vi "CD Read Engine_Simulate Records.vi"(8 "error in (no error)":errorcluster) -> (0 "error out":errorcluster, 3 "Record []":T1[](array[typedef]) {"type" format="%04x"; "activity" format="%04x"; "error" format="%04x"; "cwd1" format="%04x"; "cwd2" format="%04x"; "swd1" format="%04x"; "swd2" format="%04x"; "data" format="%04x"})   [LabVIEW 2017, in "Ballard MIL-1553 Engine.lvlib"]
uses:
  Ballard MIL-1553 Engine.lvlib
  <instrlib>/BTICardLib/Public/Controls/1553 Record.ctl
  <instrlib>/BTICardLib/BTICardLV.lvlib
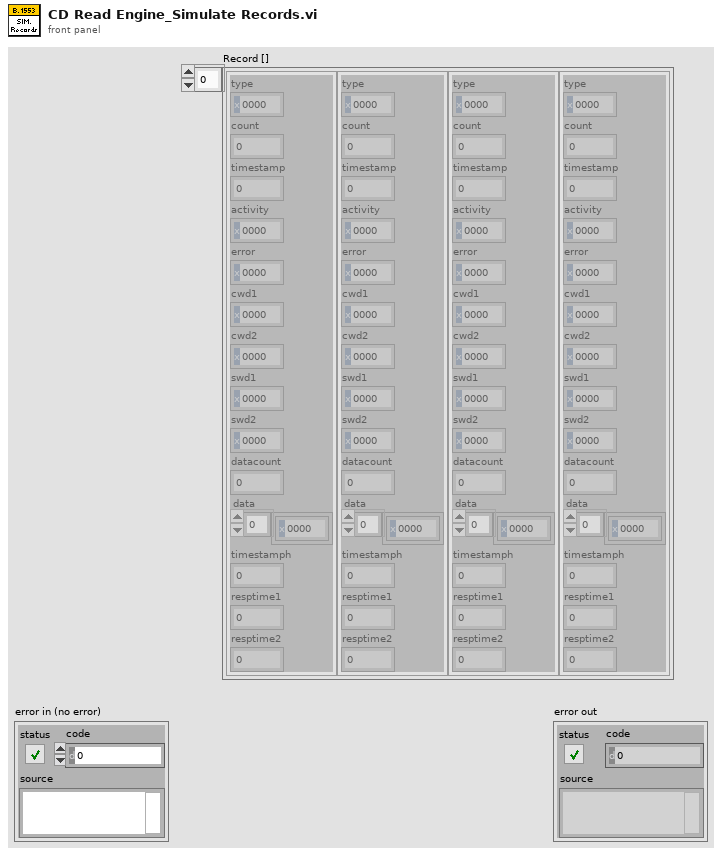
[diagram p1: front panel]
types:
  T1 = typedef "BTICardLV.lvlib/1553 Record.ctl" = cluster{"type":u16, "count":u16, "timestamp":u32, "activity":u16, "error":u16, "cwd1":u16, "cwd2":u16, "swd1":u16, "swd2":u16, "datacount":u16, "data":u16[], "timestamph":u32, "resptime1":u16, "resptime2":u16}
  T2 = cluster{"type":u16, "count":i32, "timestamp":u32, "activity":i32, "error":u16, "cwd1":i32, "cwd2":i32, "swd1":i32, "swd2":i32, "datacount":i32, "data":u16[], "timestamph":u32, "resptime1":u16, "resptime2":u16}
  T3 = cluster{"type":u16, "count":i32, "timestamp":u32, "activity":i32, "error":u16, "cwd1":i32, "cwd2":i32, "swd1":i32, "swd2":i32, "datacount":i32, "data":u16[], "timestamph":u32, "resptime1":u16, "resptime2":u16}[]
  T4 = cluster{"type":u16, "count":i32, "timestamp":u32, "activity":i32, "error":u16, "cwd1":i32, "cwd2":i32, "swd1":u16, "swd2":i32, "datacount":i32, "data":u16[], "timestamph":u32, "resptime1":u16, "resptime2":u16}
  T5 = cluster{"type":u16, "count":i32, "timestamp":u32, "activity":i32, "error":u16, "cwd1":i32, "cwd2":i32, "swd1":u16, "swd2":i32, "datacount":i32, "data":u16[], "timestamph":u32, "resptime1":u16, "resptime2":u16}[]
  T6 = cluster{"type":u16, "count":i32, "timestamp":u32, "activity":i32, "error":i32, "cwd1":i32, "cwd2":i32, "swd1":u16, "swd2":i32, "datacount":i32, "data":u16[], "timestamph":u32, "resptime1":u16, "resptime2":u16}
  T7 = cluster{"type":u16, "count":i32, "timestamp":u32, "activity":i32, "error":i32, "cwd1":i32, "cwd2":i32, "swd1":u16, "swd2":i32, "datacount":i32, "data":u16[], "timestamph":u32, "resptime1":u16, "resptime2":u16}[]
  T8 = cluster{"type":u16, "count":i32, "timestamp":u32, "activity":i32, "error":i32, "cwd1":i32, "cwd2":i32, "swd1":i32, "swd2":i32, "datacount":i32, "data":u16[], "timestamph":u32, "resptime1":u16, "resptime2":u16}[]
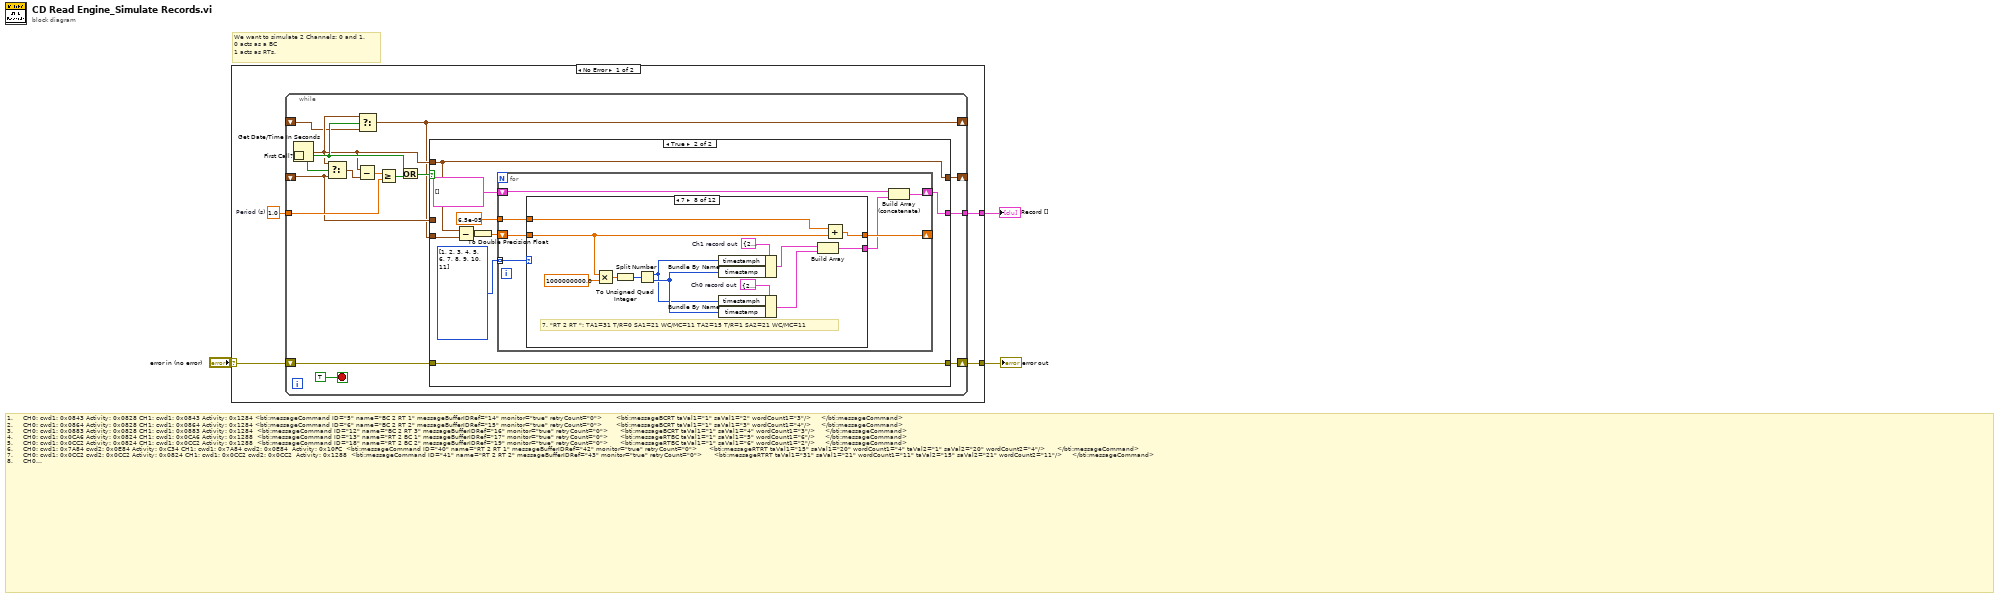
[diagram p0: block diagram]
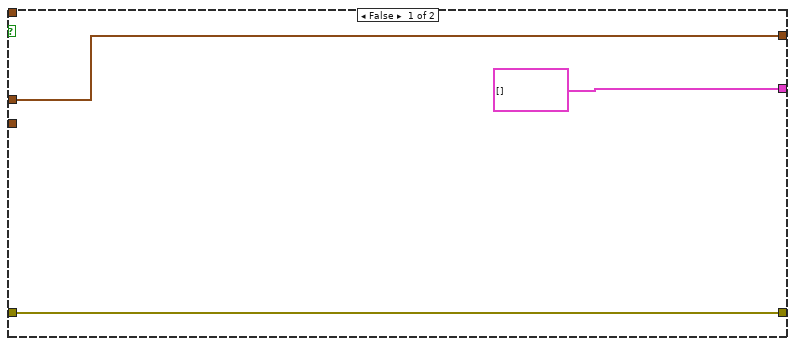
[diagram p2: hidden frame]
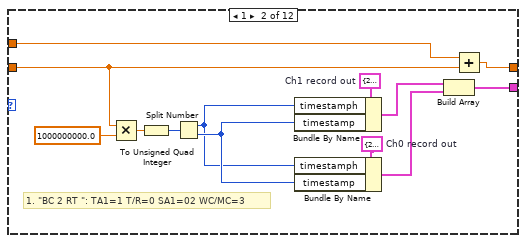
[diagram p4: hidden frame]
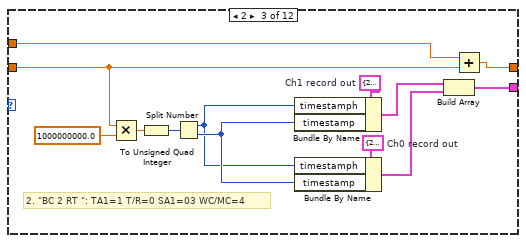
[diagram p5: hidden frame]
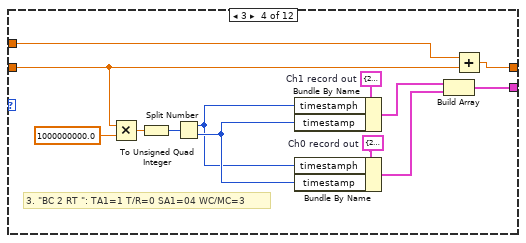
[diagram p6: hidden frame]
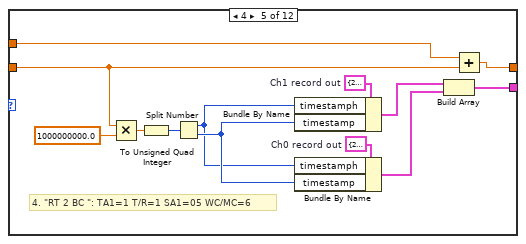
[diagram p7: hidden frame]
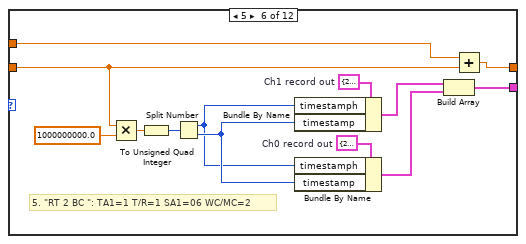
[diagram p8: hidden frame]
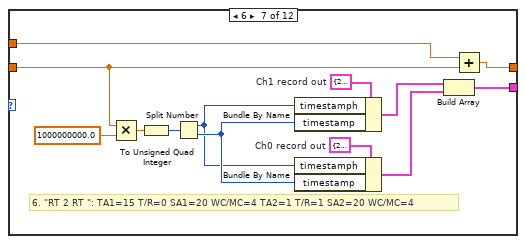
[diagram p9: hidden frame]
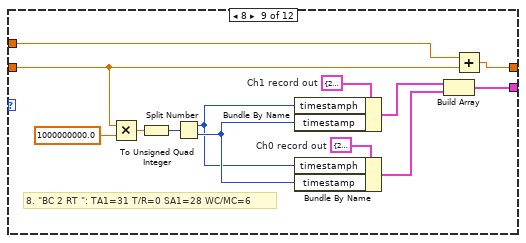
[diagram p10: hidden frame]
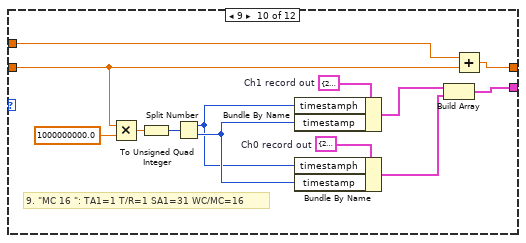
[diagram p11: hidden frame]
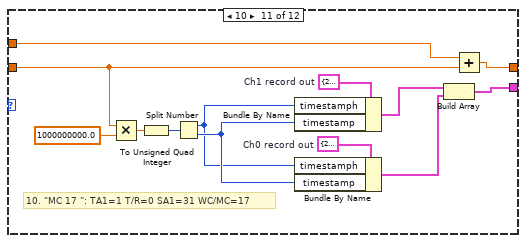
[diagram p12: hidden frame]
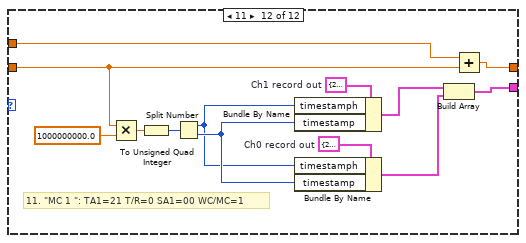
[diagram p13: hidden frame]
diagram:
  # "1.\t\t\t\t\tCH0: cwd1: 0x0843 Activity: 0x0828 CH1: cwd1: 0x0843 Activity: 0x1284 <bti:messageCommand ID=\"5\" name=\"BC 2 RT 1\" messageBufferIDRef=\"14\" monitor=\"true\" retryCount=\"0\"> \t\t\t\t\t\t<bti:messageBCRT taVal1=\"1\" saVal1=\"2\" wordCount1=\"3\"/>\t\t\t\t\t</bti:messageCommand>\n2.\t\t\t\t CH0: cwd1: 0x0864 Activity: 0x0828 CH1: cwd1: 0x0864 Activity: 0x1284 <bti:messageCommand ID=\"6\" name=\"BC 2 RT 2\" messageBufferIDRef=\"15\" monitor=\"true\" retryCount=\"0\"> \t\t\t\t\t\t<bti:messageBCRT taVal1=\"1\" saVal1=\"3\" wordCount1=\"4\"/>\t\t\t\t\t</bti:messageCommand>\n3.\t\t\t\t CH0: cwd1: 0x0883 Activity: 0x0828 CH1: cwd1: 0x0883 Activity: 0x1284 \t<bti:messageCommand ID=\"12\" name=\"BC 2 RT 3\" messageBufferIDRef=\"16\" monitor=\"true\" retryCount=\"0\">\t\t\t\t\t\t<bti:messageBCRT taVal1=\"1\" saVal1=\"4\" wordCount1=\"3\"/>\t\t\t\t\t</bti:messageCommand>\n4.\t\t\t\t\tCH0: cwd1: 0x0CA6 Activity: 0x0824 CH1: cwd1: 0x0CA6 Activity: 0x1288 \t<bti:messageCommand ID=\"13\" name=\"RT 2 BC 1\" messageBufferIDRef=\"17\" monitor=\"true\" retryCount=\"0\">\t\t\t\t\t\t<bti:messageRTBC taVal1=\"1\" saVal1=\"5\" wordCount1=\"6\"/>\t\t\t\t\t</bti:messageCommand>\n5.\t\t\t\t\tCH0: cwd1: 0x0CC2 Activity: 0x0824 CH1: cwd1: 0x0CC2 Activity: 0x1288 \t<bti:messageCommand ID=\"18\" name=\"RT 2 BC 2\" messageBufferIDRef=\"19\" monitor=\"true\" retryCount=\"0\">\t\t\t\t\t\t<bti:messageRTBC taVal1=\"1\" saVal1=\"6\" wordCount1=\"2\"/>\t\t\t\t\t</bti:messageCommand>\n6.\t\t\t\t\tCH0: cwd1: 0x7A84 cwd2: 0x0E84 Activity: 0xC34 CH1: cwd1: 0x7A84 cwd2: 0x0E84  Activity: 0x10FC \t<bti:messageCommand ID=\"40\" name=\"RT 2 RT 1\" messageBufferIDRef=\"42\" monitor=\"true\" retryCount=\"0\">\t\t\t\t\t\t<bti:messageRTRT taVal1=\"15\" saVal1=\"20\" wordCount1=\"4\" taVal2=\"1\" saVal2=\"20\" wordCount2=\"4\"/> \t\t\t\t\t</bti:messageCommand>\n7.\t\t\t\t\tCH0: cwd1: 0x0CC2 cwd2: 0x0CC2 Activity: 0x0824 CH1: cwd1: 0x0CC2 cwd2: 0x0CC2  Activity: 0x1288 \t<bti:messageCommand ID=\"41\" name=\"RT 2 RT 2\" messageBufferIDRef=\"43\" monitor=\"true\" retryCount=\"0\">\t\t\t\t\t\t<bti:messageRTRT taVal1=\"31\" saVal1=\"21\" wordCount1=\"11\" taVal2=\"15\" saVal2=\"21\" wordCount2=\"11\"/>\t\t\t\t\t</bti:messageCommand>\n8.\t\t\t\t\tCH0: cwd1: 0xFB86 Activity: 0x0808 CH1: cwd1: 0xFB86 Activity: 0x1084 <bti:messageCommand ID=\"44\" name=\"BC 2 RT 4\" messageBufferIDRef=\"45\" monitor=\"true\" retryCount=\"0\">\t\t\t\t\t\t<bti:messageBCRT taVal1=\"31\" saVal1=\"28\" wordCount1=\"6\"/> \t\t\t\t\t</bti:messageCommand>\n9.\t\t\t\t\tCH0: cwd1: 0x0FE1 Activity: 0x820 CH1: cwd1: 0x0FE1 Activity: 0x1280 <bti:messageCommand ID=\"50\" name=\"MC 16\" messageBufferIDRef=\"53\" monitor=\"true\" retryCount=\"0\">\t\t\t\t\t\t<bti:messageMC taVal1=\"1\" saVal1=\"31\" modeCodeNumber=\"16\" direction=\"Tx\"/>\t\t\t\t\t</bti:messageCommand>\n10.\t\t\tCH0: cwd1: 0x0BF1 Activity: 0x0828 CH1: cwd1: 0x0BF1 Activity: 0x1284\t\t<bti:messageCommand ID=\"51\" name=\"MC 17\" messageBufferIDRef=\"54\" monitor=\"true\" retryCount=\"0\">\t\t\t\t\t\t<bti:messageMC taVal1=\"1\" saVal1=\"31\" modeCodeNumber=\"17\" direction=\"Rx\"/>\t\t\t\t\t</bti:messageCommand>\n11.\t\t\tCH0: cwd1: 0xA801 Activity: 0x1280 CH1: cwd1:A801 0x Activity: 0x0820\t\t<bti:messageCommand ID=\"52\" name=\"MC 1\" messageBufferIDRef=\"55\" monitor=\"true\" retryCount=\"0\">\t\t\t\t\t\t<bti:messageMC taVal1=\"21\" saVal1=\"00\" modeCodeNumber=\"1\" direction=\"Rx\"/>\t\t\t\t\t</bti:messageCommand>"
  # "We want to simulate 2 Channels: 0 and 1.\n0 acts as a BC\n1 acts as RTs."
  n1 = case shown="No Error" "error in (no error)" {
    selector: "error in (no error)" -> [w7 w186]
    tunnel: [w6 w186] -> w2
    tunnel: [w4 _] -> w1
    frame No Error {
      w5 = 1.0  # Period (s)
      n2 = while {
        shift-right: [w15] -> w6
        shift-left: w7 -> [w16]
        shift-right: [w12] -> _
        shift-left: _ -> [w13]
        tunnel: w5 -> [w19]
        tunnel: [w14] -> w4
        shift-right: [w8] -> _
        shift-left: _ -> [w9]
        stop <- TRUE stop-if-true
        n3 = First Call?() -> (First Call?: T/F=w11:bool)
        n4 = Get Date/Time In Seconds() -> (seconds since 1Jan1904=w10:timestamp)
        n5 = Select(t=w10, s=w11, f=w13) -> (s? t:f=w21:timestamp)
        n6 = Subtract(x=w10, y=w21) -> (x-y=w20:dbl)
        n7 = Select(t=w10, s=w11, f=w9) -> (s? t:f=w8:timestamp)
        n8 = Greater Or Equal?(x=w20, y=w19) -> (x >= y?=w18:bool)
        n9 = Or(x=w11, y=w18) -> (x .or. y?=w17:bool)
        n10 = case shown="True" w17 {
          tunnel: w16 -> [w25 w34]
          tunnel: [w25 w34] -> w15
          tunnel: [T1[] [] ("Record []") w28] -> w14
          tunnel: w10 -> [_ w32]
          tunnel: w13 -> [w23 _]
          tunnel: [w23 w32] -> w12
          tunnel: w8 -> [_ w33]
          frame False {
          }
          frame True {
            n11 = Subtract(x=w32, y=w33) -> (x-y=w30:dbl)
            n12 = To Double Precision Float(number=w30) -> (double precision float=w31:dbl)
            n13 = for {
              shift-right: [w36] -> _
              shift-left: w31 -> [w38]
              tunnel: u8[] [1, 2, 3, 4, 5, 6, 7, 8, 9, 10, 11] -> [w39] mode=indexing
              shift-right: [w40] -> w28
              shift-left: T1[] [] ("Record []") -> [w41]
              tunnel: 6.5e-05 -> [w37]
              n14 = case shown="7" w39 {
                tunnel: w38 -> [w42 w47 w60 w73 w86 w99 w112 w125 w138 w152 w165 w178]
                tunnel: w37 -> [_ w55 w68 w81 w94 w107 w120 w133 w146 w159 w172 w185]
                tunnel: [w42 w54 w67 w80 w93 w106 w119 w132 w145 w158 w171 w184] -> w36
                tunnel: [_ w45 w59 w72 w85 w98 w111 w124 w136 w151 w164 w177] -> w35
                frame 0, Default {
                }
                frame 1 {
                  w43 = T2 {"type"=259, "count"=18, "timestamp"=1960777256, "activity"=2088, "error"=1, "cwd1"=2115, "cwd2"=0, "swd1"=30721, "swd2"=0, "datacount"=3, "data"=[1, 2, 3], "timestamph"=24, "resptime1"=87, "resptime2"=88}  # Ch0 record out
                  w44 = T2 {"type"=259, "count"=18, "timestamp"=1960777756, "activity"=4740, "error"=1, "cwd1"=2115, "cwd2"=0, "swd1"=30721, "swd2"=0, "datacount"=3, "data"=[1, 2, 3], "timestamph"=24, "resptime1"=90, "resptime2"=90}  # Ch1 record out
                  # "1. \"BC 2 RT \": TA1=1 T/R=0 SA1=02 WC/MC=3"
                  n15 = Multiply(x=w47, y=1000000000.0) -> (x*y=w51:dbl)
                  n16 = To Unsigned Quad Integer(1:w51) -> (0:w50:u64)
                  n17 = Split Number(x=w50) -> (hi(x)=w48:u32, lo(x)=w49:u32)
                  n18 = Bundle By Name(cluster=w44, "timestamph"=w48, "timestamp"=w49) -> (w46:T2)
                  n19 = Bundle By Name(cluster=w43, "timestamph"=w48, "timestamp"=w49) -> (w53:T2)
                  n20 = Build Array(w46, w53) -> (w45:T3)
                  n21 = Add(x=w55, y=w47) -> (x+y=w54:dbl)
                }
                frame 2 {
                  w56 = T2 {"type"=259, "count"=19, "timestamp"=1960777256, "activity"=2088, "error"=1, "cwd1"=2148, "cwd2"=0, "swd1"=30721, "swd2"=0, "datacount"=4, "data"=[4, 5, 6, 7], "timestamph"=24, "resptime1"=87, "resptime2"=88}  # Ch0 record out
                  w57 = T2 {"type"=259, "count"=19, "timestamp"=1960777756, "activity"=4740, "error"=1, "cwd1"=2148, "cwd2"=0, "swd1"=30721, "swd2"=0, "datacount"=4, "data"=[4, 5, 6, 7], "timestamph"=24, "resptime1"=90, "resptime2"=90}  # Ch1 record out
                  # "2. \"BC 2 RT \": TA1=1 T/R=0 SA1=03 WC/MC=4"
                  n22 = Multiply(x=w60, y=1000000000.0) -> (x*y=w64:dbl)
                  n23 = To Unsigned Quad Integer(1:w64) -> (0:w63:u64)
                  n24 = Split Number(x=w63) -> (hi(x)=w61:u32, lo(x)=w62:u32)
                  n25 = Bundle By Name(cluster=w57, "timestamph"=w61, "timestamp"=w62) -> (w58:T2)
                  n26 = Bundle By Name(cluster=w56, "timestamph"=w61, "timestamp"=w62) -> (w66:T2)
                  n27 = Build Array(w58, w66) -> (w59:T3)
                  n28 = Add(x=w68, y=w60) -> (x+y=w67:dbl)
                }
                frame 3 {
                  w69 = T2 {"type"=259, "count"=18, "timestamp"=1960777256, "activity"=2088, "error"=1, "cwd1"=2179, "cwd2"=0, "swd1"=30721, "swd2"=0, "datacount"=3, "data"=[8, 9, 10], "timestamph"=24, "resptime1"=87, "resptime2"=88}  # Ch0 record out
                  w70 = T2 {"type"=259, "count"=18, "timestamp"=1960777756, "activity"=4740, "error"=1, "cwd1"=2179, "cwd2"=0, "swd1"=30721, "swd2"=0, "datacount"=3, "data"=[8, 9, 10], "timestamph"=24, "resptime1"=90, "resptime2"=90}  # Ch1 record out
                  # "3. \"BC 2 RT \": TA1=1 T/R=0 SA1=04 WC/MC=3"
                  n29 = Multiply(x=w73, y=1000000000.0) -> (x*y=w77:dbl)
                  n30 = To Unsigned Quad Integer(1:w77) -> (0:w76:u64)
                  n31 = Split Number(x=w76) -> (hi(x)=w74:u32, lo(x)=w75:u32)
                  n32 = Bundle By Name(cluster=w70, "timestamph"=w74, "timestamp"=w75) -> (w71:T2)
                  n33 = Bundle By Name(cluster=w69, "timestamph"=w74, "timestamp"=w75) -> (w79:T2)
                  n34 = Build Array(w71, w79) -> (w72:T3)
                  n35 = Add(x=w81, y=w73) -> (x+y=w80:dbl)
                }
                frame 4 {
                  w82 = T4 {"type"=259, "count"=21, "timestamp"=1960777256, "activity"=2084, "error"=1, "cwd1"=3238, "cwd2"=0, "swd1"=30720, "swd2"=0, "datacount"=6, "data"=[11, 12, 13, 14, 15, 16], "timestamph"=24, "resptime1"=87, "resptime2"=88}  # Ch0 record out
                  w83 = T4 {"type"=259, "count"=21, "timestamp"=1960777756, "activity"=4744, "error"=1, "cwd1"=3238, "cwd2"=0, "swd1"=30720, "swd2"=0, "datacount"=6, "data"=[11, 12, 13, 14, 15, 16], "timestamph"=24, "resptime1"=90, "resptime2"=90}  # Ch1 record out
                  # "4. \"RT 2 BC \": TA1=1 T/R=1 SA1=05 WC/MC=6"
                  n36 = Multiply(x=w86, y=1000000000.0) -> (x*y=w90:dbl)
                  n37 = To Unsigned Quad Integer(1:w90) -> (0:w89:u64)
                  n38 = Split Number(x=w89) -> (hi(x)=w87:u32, lo(x)=w88:u32)
                  n39 = Bundle By Name(cluster=w83, "timestamph"=w87, "timestamp"=w88) -> (w84:T4)
                  n40 = Bundle By Name(cluster=w82, "timestamph"=w87, "timestamp"=w88) -> (w92:T4)
                  n41 = Build Array(w84, w92) -> (w85:T5)
                  n42 = Add(x=w94, y=w86) -> (x+y=w93:dbl)
                }
                frame 5 {
                  w95 = T4 {"type"=259, "count"=17, "timestamp"=1960777256, "activity"=2084, "error"=1, "cwd1"=3266, "cwd2"=0, "swd1"=30720, "swd2"=0, "datacount"=2, "data"=[17, 18], "timestamph"=24, "resptime1"=87, "resptime2"=88}  # Ch0 record out
                  w96 = T4 {"type"=259, "count"=17, "timestamp"=1960777756, "activity"=4744, "error"=1, "cwd1"=3266, "cwd2"=0, "swd1"=30720, "swd2"=0, "datacount"=2, "data"=[17, 18], "timestamph"=24, "resptime1"=90, "resptime2"=90}  # Ch1 record out
                  # "5. \"RT 2 BC \": TA1=1 T/R=1 SA1=06 WC/MC=2"
                  n43 = Multiply(x=w99, y=1000000000.0) -> (x*y=w103:dbl)
                  n44 = To Unsigned Quad Integer(1:w103) -> (0:w102:u64)
                  n45 = Split Number(x=w102) -> (hi(x)=w100:u32, lo(x)=w101:u32)
                  n46 = Bundle By Name(cluster=w96, "timestamph"=w100, "timestamp"=w101) -> (w97:T4)
                  n47 = Bundle By Name(cluster=w95, "timestamph"=w100, "timestamp"=w101) -> (w105:T4)
                  n48 = Build Array(w97, w105) -> (w98:T5)
                  n49 = Add(x=w107, y=w99) -> (x+y=w106:dbl)
                }
                frame 6 {
                  w108 = T6 {"type"=259, "count"=19, "timestamp"=1960777256, "activity"=3124, "error"=1, "cwd1"=31364, "cwd2"=3716, "swd1"=30720, "swd2"=30721, "datacount"=4, "data"=[19, 20, 21, 22], "timestamph"=24, "resptime1"=87, "resptime2"=88}  # Ch0 record out
                  w109 = T6 {"type"=259, "count"=19, "timestamp"=1960777756, "activity"=4348, "error"=1, "cwd1"=31364, "cwd2"=3716, "swd1"=30720, "swd2"=30721, "datacount"=4, "data"=[19, 20, 21, 22], "timestamph"=24, "resptime1"=90, "resptime2"=90}  # Ch1 record out
                  # "6. \"RT 2 RT \": TA1=15 T/R=0 SA1=20 WC/MC=4 TA2=1 T/R=1 SA2=20 WC/MC=4"
                  n50 = Multiply(x=w112, y=1000000000.0) -> (x*y=w116:dbl)
                  n51 = To Unsigned Quad Integer(1:w116) -> (0:w115:u64)
                  n52 = Split Number(x=w115) -> (hi(x)=w113:u32, lo(x)=w114:u32)
                  n53 = Bundle By Name(cluster=w109, "timestamph"=w113, "timestamp"=w114) -> (w110:T6)
                  n54 = Bundle By Name(cluster=w108, "timestamph"=w113, "timestamp"=w114) -> (w118:T6)
                  n55 = Build Array(w110, w118) -> (w111:T7)
                  n56 = Add(x=w120, y=w112) -> (x+y=w119:dbl)
                }
                frame 7 {
                  w121 = T6 {"type"=259, "count"=26, "timestamp"=1960777756, "activity"=4300, "error"=32769, "cwd1"=64171, "cwd2"=32427, "swd1"=30720, "swd2"=30721, "datacount"=11, "data"=[522, 523, 524, 525, 526, 527, 528, 529, 530, 531, 532], "timestamph"=24, "resptime1"=90, "resptime2"=90}  # Ch1 record out
                  w122 = T6 {"type"=259, "count"=26, "timestamp"=1960777256, "activity"=3076, "error"=32769, "cwd1"=64171, "cwd2"=32427, "swd1"=30720, "swd2"=30721, "datacount"=11, "data"=[522, 523, 524, 525, 526, 527, 528, 529, 530, 531, 532], "timestamph"=24, "resptime1"=87, "resptime2"=88}  # Ch0 record out
                  # "7. \"RT 2 RT \": TA1=31 T/R=0 SA1=21 WC/MC=11 TA2=15 T/R=1 SA2=21 WC/MC=11"
                  n57 = Multiply(x=w125, y=1000000000.0) -> (x*y=w129:dbl)
                  n58 = To Unsigned Quad Integer(1:w129) -> (0:w128:u64)
                  n59 = Split Number(x=w128) -> (hi(x)=w126:u32, lo(x)=w127:u32)
                  n60 = Bundle By Name(cluster=w121, "timestamph"=w126, "timestamp"=w127) -> (w123:T6)
                  n61 = Bundle By Name(cluster=w122, "timestamph"=w126, "timestamp"=w127) -> (w131:T6)
                  n62 = Build Array(w123, w131) -> (w124:T7)
                  n63 = Add(x=w133, y=w125) -> (x+y=w132:dbl)
                }
                frame 8 {
                  w134 = T2 {"type"=259, "count"=21, "timestamp"=1960777756, "activity"=4228, "error"=1, "cwd1"=64390, "cwd2"=0, "swd1"=0, "swd2"=0, "datacount"=6, "data"=[49, 50, 51, 52, 53, 54], "timestamph"=24, "resptime1"=90, "resptime2"=90}  # Ch1 record out
                  w135 = T2 {"type"=259, "count"=21, "timestamp"=1960777256, "activity"=2056, "error"=1, "cwd1"=64390, "cwd2"=0, "swd1"=0, "swd2"=0, "datacount"=6, "data"=[49, 50, 51, 52, 53, 54], "timestamph"=24, "resptime1"=87, "resptime2"=88}  # Ch0 record out
                  # "8. \"BC 2 RT \": TA1=31 T/R=0 SA1=28 WC/MC=6"
                  n64 = Multiply(x=w138, y=1000000000.0) -> (x*y=w142:dbl)
                  n65 = To Unsigned Quad Integer(1:w142) -> (0:w141:u64)
                  n66 = Split Number(x=w141) -> (hi(x)=w139:u32, lo(x)=w140:u32)
                  n67 = Bundle By Name(cluster=w134, "timestamph"=w139, "timestamp"=w140) -> (w137:T2)
                  n68 = Bundle By Name(cluster=w135, "timestamph"=w139, "timestamp"=w140) -> (w144:T2)
                  n69 = Build Array(w137, w144) -> (w136:T3)
                  n70 = Add(x=w146, y=w138) -> (x+y=w145:dbl)
                }
                frame 9 {
                  w147 = T2 {"type"=259, "count"=16, "timestamp"=1960777256, "activity"=2084, "error"=1, "cwd1"=4080, "cwd2"=0, "swd1"=32720, "swd2"=0, "datacount"=1, "data"=[65244], "timestamph"=24, "resptime1"=87, "resptime2"=88}  # Ch0 record out
                  w148 = T2 {"type"=259, "count"=16, "timestamp"=1960777756, "activity"=4744, "error"=1, "cwd1"=4080, "cwd2"=0, "swd1"=32720, "swd2"=0, "datacount"=1, "data"=[65244], "timestamph"=24, "resptime1"=90, "resptime2"=90}  # Ch1 record out
                  # "9. \"MC 16 \": TA1=1 T/R=1 SA1=31 WC/MC=16"
                  n71 = Multiply(x=w152, y=1000000000.0) -> (x*y=w156:dbl)
                  n72 = To Unsigned Quad Integer(1:w156) -> (0:w155:u64)
                  n73 = Split Number(x=w155) -> (hi(x)=w153:u32, lo(x)=w154:u32)
                  n74 = Bundle By Name(cluster=w148, "timestamph"=w153, "timestamp"=w154) -> (w150:T2)
                  n75 = Bundle By Name(cluster=w147, "timestamph"=w153, "timestamp"=w154) -> (w149:T2)
                  n76 = Build Array(w150, w149) -> (w151:T3)
                  n77 = Add(x=w159, y=w152) -> (x+y=w158:dbl)
                }
                frame 10 {
                  w160 = T2 {"type"=259, "count"=16, "timestamp"=1960777756, "activity"=4744, "error"=1, "cwd1"=3057, "cwd2"=0, "swd1"=32720, "swd2"=0, "datacount"=1, "data"=[20736], "timestamph"=24, "resptime1"=90, "resptime2"=90}  # Ch1 record out
                  w161 = T2 {"type"=259, "count"=16, "timestamp"=1960777256, "activity"=2088, "error"=1, "cwd1"=3057, "cwd2"=0, "swd1"=32720, "swd2"=0, "datacount"=1, "data"=[20736], "timestamph"=24, "resptime1"=87, "resptime2"=88}  # Ch0 record out
                  # "10. \"MC 17 \": TA1=1 T/R=0 SA1=31 WC/MC=17"
                  n78 = Multiply(x=w165, y=1000000000.0) -> (x*y=w169:dbl)
                  n79 = To Unsigned Quad Integer(1:w169) -> (0:w168:u64)
                  n80 = Split Number(x=w168) -> (hi(x)=w166:u32, lo(x)=w167:u32)
                  n81 = Bundle By Name(cluster=w160, "timestamph"=w166, "timestamp"=w167) -> (w163:T2)
                  n82 = Bundle By Name(cluster=w161, "timestamph"=w166, "timestamp"=w167) -> (w162:T2)
                  n83 = Build Array(w163, w162) -> (w164:T3)
                  n84 = Add(x=w172, y=w165) -> (x+y=w171:dbl)
                }
                frame 11 {
                  w173 = T2 {"type"=259, "count"=15, "timestamp"=1960777256, "activity"=2080, "error"=1, "cwd1"=43009, "cwd2"=0, "swd1"=32720, "swd2"=0, "datacount"=0, "data"=[], "timestamph"=24, "resptime1"=87, "resptime2"=88}  # Ch0 record out
                  w174 = T2 {"type"=259, "count"=15, "timestamp"=1960777756, "activity"=4736, "error"=1, "cwd1"=43009, "cwd2"=0, "swd1"=32720, "swd2"=0, "datacount"=0, "data"=[], "timestamph"=24, "resptime1"=90, "resptime2"=90}  # Ch1 record out
                  # "11. \"MC 1 \": TA1=21 T/R=0 SA1=00 WC/MC=1"
                  n85 = Multiply(x=w178, y=1000000000.0) -> (x*y=w182:dbl)
                  n86 = To Unsigned Quad Integer(1:w182) -> (0:w181:u64)
                  n87 = Split Number(x=w181) -> (hi(x)=w179:u32, lo(x)=w180:u32)
                  n88 = Bundle By Name(cluster=w174, "timestamph"=w179, "timestamp"=w180) -> (w176:T2)
                  n89 = Bundle By Name(cluster=w173, "timestamph"=w179, "timestamp"=w180) -> (w175:T2)
                  n90 = Build Array(w176, w175) -> (w177:T3)
                  n91 = Add(x=w185, y=w178) -> (x+y=w184:dbl)
                }
              }
              n92 = Build Array (concatenate)(w41, w35) -> (w40:T8)
            }
          }
        }
      }
    }
    frame Error {
    }
  }
  "Record []" <- w1
  "error out" <- w2
